vi "launch alice and bob.vi"() -> ()   [LabVIEW 2014]
uses:
  Bob/Bob/Bob.lvclass
  Network Stream Reader/Network Stream Reader/Network Stream Reader.lvclass
  Alice/Alice/Alice.lvclass
  Network Stream Writer/Network Stream Writer/Network Stream Writer.lvclass
  Alice/Alice Messages/Proceed failed Msg Msg/Proceed failed Msg Msg.lvclass
  Alice/Alice Messages/Proceed connection state Msg/Proceed connection state Msg.lvclass
  Proxy/Proxy/Proxy.lvclass/Proxy.ctl
  Network Stream/Network Stream/Network Stream.lvclass/Network Stream.ctl
  Alice/Alice Messages/Write Bob Enq Msg/Write Bob Enq Msg.lvclass/Write Bob Enq Msg.ctl
  <vilib>/ActorFramework/Message Enqueuer/Message Enqueuer.lvclass/Message Enqueuer.ctl
  Proxy/Proxy/Write Target Enq.vi
  Network Stream/Network Stream/Write Context.vi
  Network Stream/Network Stream/Write Name.vi
  Proxy/Proxy/Write Return Message Msg.vi
  Proxy/Proxy/Write Status Msg.vi
  <vilib>/ActorFramework/Message Enqueuer/Enqueue.vi
  <vilib>/ActorFramework/Message Priority Queue/Priority Enqueue.vi
  Alice/Alice Messages/Write Bob Enq Msg/Write Bob Enq Msg.lvclass
  <vilib>/ActorFramework/Stop Msg/Stop Msg.lvclass
  <vilib>/ActorFramework/Actor/Actor.lvclass
panel:
  out "error out":errorcluster
  in  "stop":bool
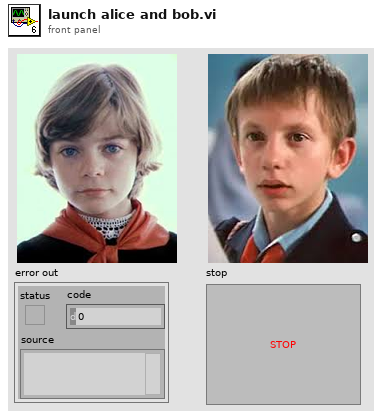
[diagram p1: front panel]
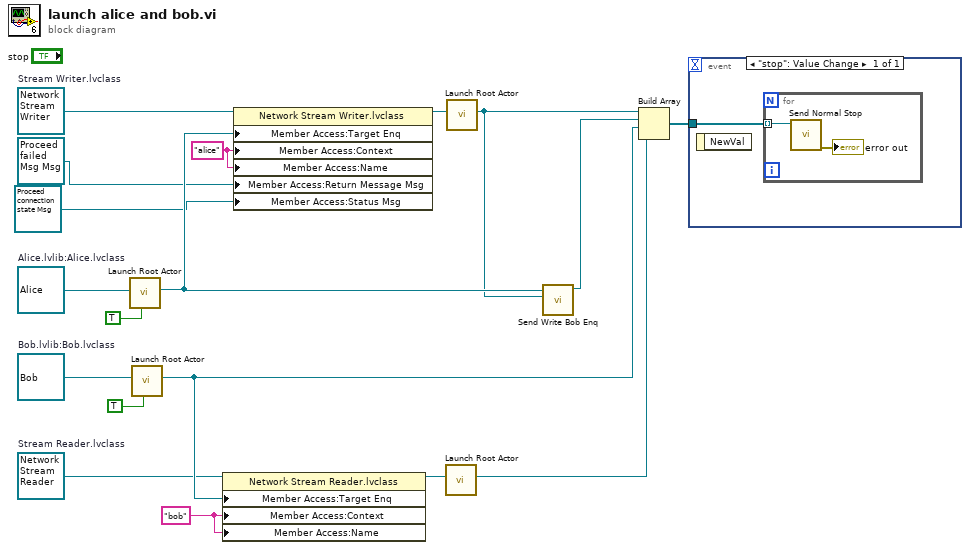
[diagram p0: block diagram]
diagram:
  w3 = "alice" ("Context")
  w6 = refnum<class "Network Stream Writer.lvclass"> refnum  # Stream Writer.lvclass
  w9 = refnum<class "Alice.lvclass"> refnum  # Alice.lvlib:Alice.lvclass
  w10 = "bob" ("Context")
  w11 = refnum<class "Network Stream Reader.lvclass"> refnum  # Stream Reader.lvclass
  w14 = refnum<class "Bob.lvclass"> refnum  # Bob.lvlib:Bob.lvclass
  n1 = call <vilib>:"Launch Root Actor.vi"("Open Actor Core front panel? (F)"=TRUE, "Actor"=w9) -> ("Actor's Enqueuer"=w7:refnum<class "Message Enqueuer.lvclass">)  [unwired: 8 in, 1 out]
  n2 = call <vilib>:"Launch Root Actor.vi"("Open Actor Core front panel? (F)"=TRUE, "Actor"=w14) -> ("Actor's Enqueuer"=w17:refnum<class "Message Enqueuer.lvclass">)  [unwired: 8 in, 1 out]
  n3 = property class="Network Stream Reader.lvclass"(reference=w11, "Member Access:Target Enq"=w17, "Member Access:Context"=w10, "Member Access:Name"=w10) -> (reference out=w12:refnum<class "Network Stream Reader.lvclass">)  [unwired: 1 in, 1 out]
  n4 = property class="Network Stream Writer.lvclass"(reference=w6, "Member Access:Target Enq"=w7, "Member Access:Context"=w3, "Member Access:Name"=w3, "Member Access:Return Message Msg"=refnum<class "Proceed failed Msg Msg.lvclass"> refnum ("Alice.lvlib:Proceed failed Msg Msg.lvclass"), "Member Access:Status Msg"=refnum<class "Proceed connection state Msg.lvclass"> refnum ("Alice.lvlib:Proceed connection state Msg.lvclass")) -> (reference out=w5:refnum<class "Network Stream Writer.lvclass">)  [unwired: 1 in, 1 out]
  n5 = call <vilib>:"Launch Root Actor.vi"("Actor"=w12) -> ("Actor's Enqueuer"=w16:refnum<class "Message Enqueuer.lvclass">)  [unwired: 9 in, 1 out]
  n6 = call <vilib>:"Launch Root Actor.vi"("Actor"=w5) -> ("Actor's Enqueuer"=w4:refnum<class "Message Enqueuer.lvclass">)  [unwired: 9 in, 1 out]
  n7 = call "Send Write Bob Enq.vi"("Actor Framework:Message Enqueuer"=w4, "Message Enqueuer"=w7) -> ("Message Enqueuer out"=w18:refnum<class "Message Enqueuer.lvclass">)  [unwired: 8 in, 1 out]
  n8 = Build Array(w4, w18, w17, w16) -> (w15:refnum<class "Message Enqueuer.lvclass">[])
  n9 = event shown="[0] \"stop\": Value Change" {
    selector: _ -> [_]
    dyn-events: _ -> [_]
    timeout: _ -> [_]
    tunnel: w15 -> [w19]
    event "stop": Value Change {
      n10 = event-data() -> ()  [unwired: 1 in, 1 out]
      n11 = for {
        tunnel: w19 -> [w21] mode=indexing
        n12 = call <vilib>:"Send Normal Stop.vi"("Message Enqueuer"=w21) -> ("error out"=→"error out":errorcluster)  [unwired: 10 in]
      }
    }
  }
